vi "ADAM_Read.vi"(8 "错误输入（无错误）":errorcluster, 11 "VISA resource name":refnum<visa-resource-name> caption="VISA资源名称") -> (0 "error out":errorcluster caption="错误输出", 1 "humidity":dbl, 2 "temperature":dbl, 3 "Data":string)   [LabVIEW 2017]
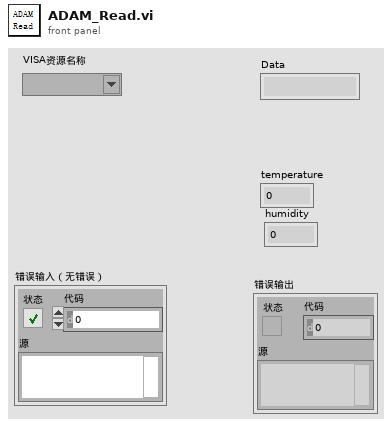
[diagram p1: front panel]
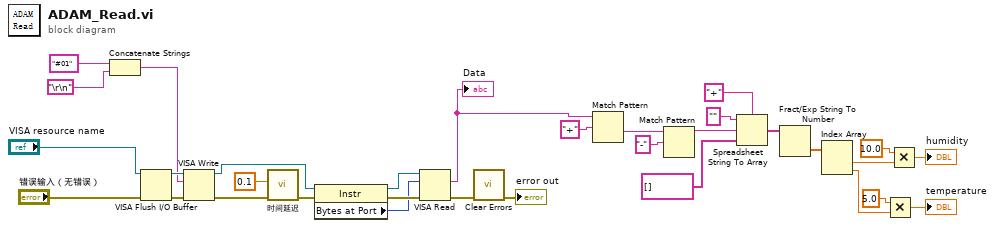
[diagram p0: block diagram]
diagram:
  n1 = Concatenate Strings("#01", "\r\n") -> (w19:string)
  n2 = VISA Flush I/O Buffer(VISA resource name="VISA resource name", error in (no error)="错误输入（无错误）") -> (VISA resource name out=w32:refnum<visa-resource-name>, error out=w30:errorcluster)  [unwired: 1 in]
  n3 = VISA Write(VISA resource name=w32, write buffer=w19, error in (no error)=w30) -> (VISA resource name out=w24:refnum<visa-resource-name>, error out=w31:errorcluster)  [unwired: 1 out]
  n4 = call "时间延迟"("error in (no error)"=w31, "Delay Time (s)"=0.1) -> ("error out"=w21:errorcluster)  [unwired: 9 in]
  n5 = property class="Instr"(reference=w24, error in=w21) -> (reference out=w23:refnum<visa-resource-name>, error out=w22:errorcluster, "Bytes at Port"=w17:u32)
  n6 = VISA Read(VISA resource name=w23, byte count=w17, error in (no error)=w22) -> (read buffer=w1:string, error out=w29:errorcluster)  [unwired: 2 out]
  "Data" <- w1
  n7 = call <vilib>:"Clear Errors.vi"("error in (no error)"=w29) -> ("error out"=→"error out":errorcluster)  [unwired: 5 in, 1 out]
  n8 = Match Pattern(string=w1, regular expression="+" ("正则表达式")) -> (after substring=w10:string)  [unwired: 1 in, 3 out]
  n9 = Match Pattern(string=w10, regular expression="-" ("正则表达式")) -> (before substring=w15:string)  [unwired: 1 in, 3 out]
  n10 = Spreadsheet String To Array(delimiter (Tab)="+" ("分隔符(Tab)"), format string="" ("格式字符串"), spreadsheet string=w15, array type (2D Dbl)=string[] []) -> (array=w9:string[])
  n11 = Fract/Exp String To Number(string=w9) -> (number=w8:dbl[])  [unwired: 3 in, 1 out]
  n12 = Index Array(array=w8) -> (element #1=w7:dbl, element #2=w4:dbl)  [unwired: 2 in]
  n13 = Multiply(x=5.0, y=w4) -> (x*y=→"temperature":dbl)
  n14 = Multiply(x=10.0, y=w7) -> (x*y=→"humidity":dbl)
